vi "Profile_Read.vi"(7 "Measurement Profile":path, 8 "error in (no error)":errorcluster, 10 "Configuration Cluster":T1={"General"={"Config.ini"=path "", "Default Logging Path"=path ""}, "Hardware"={"AHC VISA COM"="", "Measure Rate (1/s)"=0, "Global T VAR"="", "Global B VAR"=""}, "Operation"={"Operation Mode"=enum."Idle-Off", "Status"="", "NewLog?"=FALSE}}) -> (0 "error out":errorcluster, 2 "Configuration Cluster Out":T1={"General"={"Config.ini"=path "", "Default Logging Path"=path ""}, "Hardware"={"AHC VISA COM"="", "Measure Rate (1/s)"=0, "Global T VAR"="", "Global B VAR"=""}, "Operation"={"Operation Mode"=enum."Idle-Off", "Status"="", "NewLog?"=FALSE}})   [LabVIEW 2021]
uses:
  Config_Cluster.ctl
  Mode_Enum.ctl
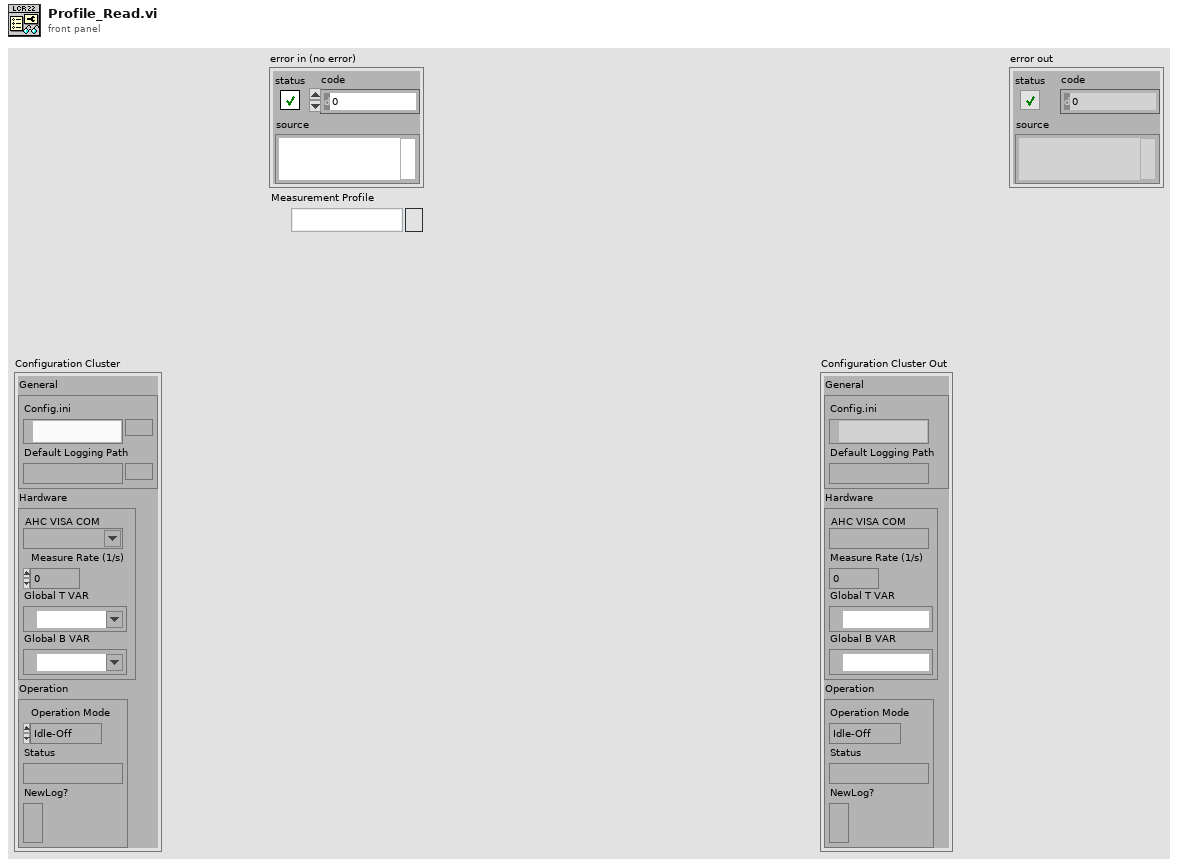
[diagram p1: front panel]
types:
  T1 = typedef "Config_Cluster.ctl" = cluster{"General":cluster{"Config.ini":path, "Default Logging Path":path}, "Hardware":cluster{"AHC VISA COM":refnum<visa-resource-name>, "Measure Rate (1/s)":i32, "Global T VAR":refnum<k21>, "Global B VAR":refnum<k21>}, "Operation":cluster{"Operation Mode":T2, "Status":string, "NewLog?":bool}}
  T2 = typedef "Mode_Enum.ctl" = enum16{"Logging", "Idle-Off", "Idle"}
  T3 = cluster{"Bias Profile":cluster{" Bias Source (OFF)":u8, " Bias Type (Voltage)":u8, "Bias Level (0)":dbl}, "Measurement Profile":cluster{"Operation Mode (0: Auto)":u16, "Circuit Type (2: Auto)":u16, "Manual Range (1:Range 1 and 25 Ohms)":u8, "Auto Range (T: Enable)":bool}, "Signal Profile":cluster{"Frequency (1kHz)":dbl, "Measuring Voltage (1V)":dbl}, "Integration Profile":cluster{"Averaging (0: Off)":u16, "Averaging Number (2)":i32, "Time (100ms)":i32, "Rate (0: Fast)":u16}, "Trigger Profile":cluster{"Trigger Mode (0: Continuous)":u16}}
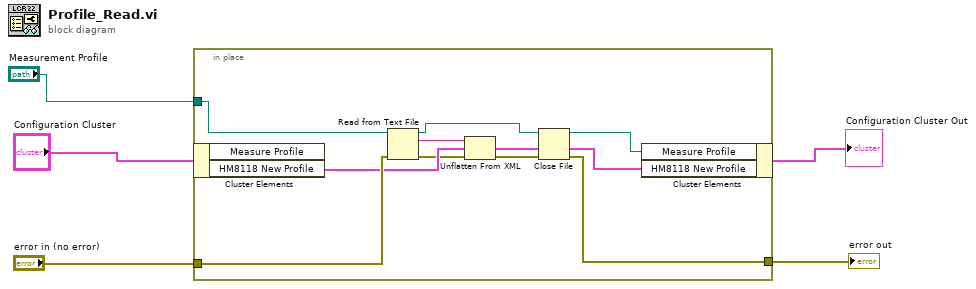
[diagram p0: block diagram]
diagram:
  n1 = in-place {
    in-place-border: "Measurement Profile" -> [w15]
    in-place-border: "error in (no error)" -> [w14]
    in-place-border: [w7] -> w1
    n2 = in-place-cluster #1("Configuration Cluster") -> ("HM8118 New Profile"=w12:T3)  [unwired: 1 out]
    n3 = Read from Text File(file (use dialog)=w15, error in=w14) -> (refnum out=w9:refnum<file>, text=w13:string, error out=w11:errorcluster)  [unwired: 2 in, 1 out]
    n4 = Unflatten From XML(xml string=w13, type=w12, error in (no error)=w11) -> (value=w10:T3, error out=w8:errorcluster)
    n5 = Close File(refnum=w9, error in=w8) -> (path=w6:path, error out=w7:errorcluster)
    n6 = in-place-cluster #1("Measure Profile"=w6, "HM8118 New Profile"=w10) -> (→"Configuration Cluster Out":T1)
  }
  "error out" <- w1
